vi "Sub03_02_ExecuteExe.vi"(8 "error in (no error)":errorcluster, 9 "String":string, 10 "vi name":string, 11 "appended path":path) -> (0 "error out":errorcluster, 2 "standard error":string, 3 "standard output":string)   [LabVIEW 2019]
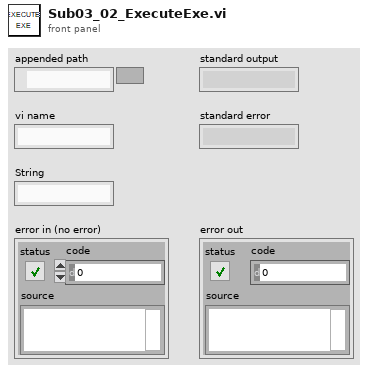
[diagram p1: front panel]
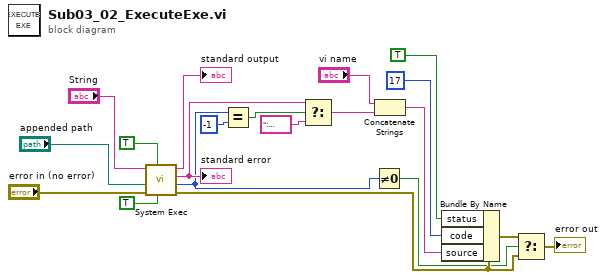
[diagram p0: block diagram]
diagram:
  n1 = call <vilib>:"System Exec.vi"("run minimized? (F)"=TRUE, "wait until completion? (T)"=TRUE, "error in (no error)"="error in (no error)", "working directory"="appended path", "command line"="String") -> ("error out"=w14:errorcluster, "return code"=w10:i32, "standard error"=w12:string, "standard output"=→"standard output":string)  [unwired: 3 in]
  "standard error" <- w12
  n2 = Equal?(x=w10, y=-1) -> (x = y?=w9:bool)
  n3 = Select(t=w12, s=w9, f=": unknown error during C execution") -> (s? t:f=w17:string)
  n4 = Not Equal To 0?(x=w10) -> (x != 0?=w8:bool)
  n5 = Concatenate Strings("vi name", w17) -> (w18:string)
  n6 = Bundle By Name(cluster=w14, "status"=TRUE, "code"=17, "source"=w18) -> (w6:errorcluster)
  n7 = Select(t=w6, s=w8, f=w14) -> (s? t:f=→"error out":errorcluster)
